vi "Exit Initialize (User).vi"(8 "error in":errorcluster, 11 "Node in":refnum<class "BLS Climate Chamber Template.lvclass">) -> (0 "error out":errorcluster, 3 "Node out":refnum<class "BLS Climate Chamber Template.lvclass">)   [LabVIEW 2023, in "BLS Climate Chamber Template.lvlib" / "BLS Climate Chamber Template.lvclass"]
uses:
  BLS Climate Chamber Template.lvclass
  C:/Program Files/National Instruments/LabVIEW 2023/vi.lib/ADAS Replay HIL/Template Node/Plugin/Template Node/Template Node.lvclass
  <vilib>/ADAS Replay HIL/Template Node/Plugin/Template Node/Template Node.lvclass/Template Node.ctl
  BLS Climate Chamber Template.lvclass/BLS Climate Chamber Template.ctl
  <vilib>/ADAS Replay HIL/Template Node/Plugin/Template Node/Template Node.lvclass
  C:/Program Files/National Instruments/ADAS Replay HIL/EVO SDK/Linux RT/evoLabVIEWAPI/evoBlockPlugin.lvlibp/evoBlockPlugin/BlockPluginInterface.2020.1/BlockPluginInterface.2020.1.lvclass
  D:/git/bls-climate-chamber-plugin-template/src/Plugin/BLS Climate Chamber Template/BLS Climate Chamber Template.lvclass
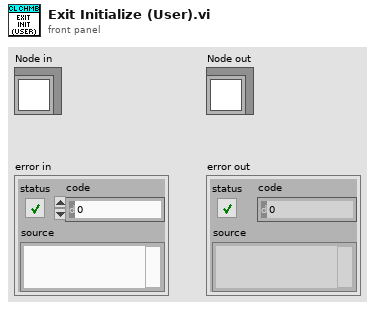
[diagram p1: front panel]
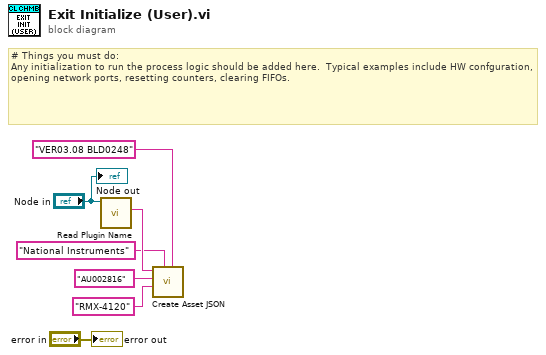
[diagram p0: block diagram]
diagram:
  # "# Things you must do:\nAny initialization to run the process logic should be added here.  Typical examples include HW confguration, opening network ports, resetting counters, clearing FIFOs."
  n1 = call <vilib>:"Read Plugin Name.vi"("Template Node in"="Node in") -> ("Plugin Name"=w6:string)  [unwired: 8 in, 2 out]
  n2 = call "Create Asset JSON.vi"("firmwareVersion"="VER03.08 BLD0248", "vendorName"="National Instruments", "modelName"="RMX-4120", "serialNumber"="AU002816", "pluginName"=w6) -> ()  [unwired: 5 in, 2 out]
  "Node out" <- "Node in"
  "error out" <- "error in"
